vi "调制信号与解调.vi"() -> ()   [LabVIEW 2018]
panel:
  out "布尔":bool
  out "数组 2":dbl[](array[numeric])
  out "解调后的波形":dynamicdata(graph)
  out "相干后时域波形":dynamicdata(graph)
  in  "停止":bool
  out "数组":dbl[](array[numeric])
  in  "垂直指针滑动杆":dbl(slide) min=0.0 max=5.0 scale=0.0..5.0
  out "波形图":dynamicdata(graph)
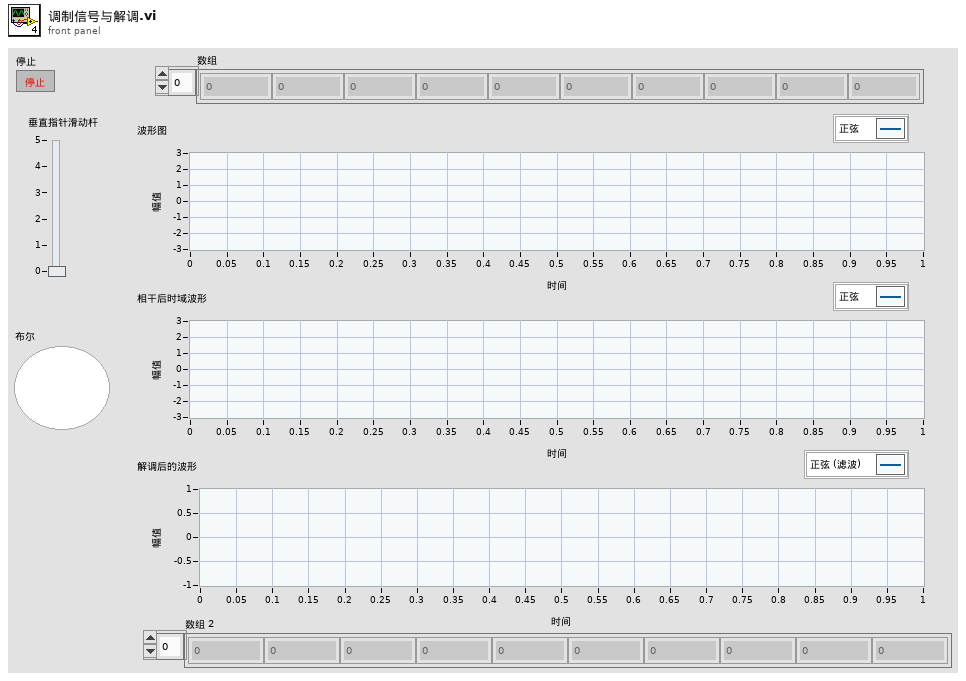
[diagram p1: front panel]
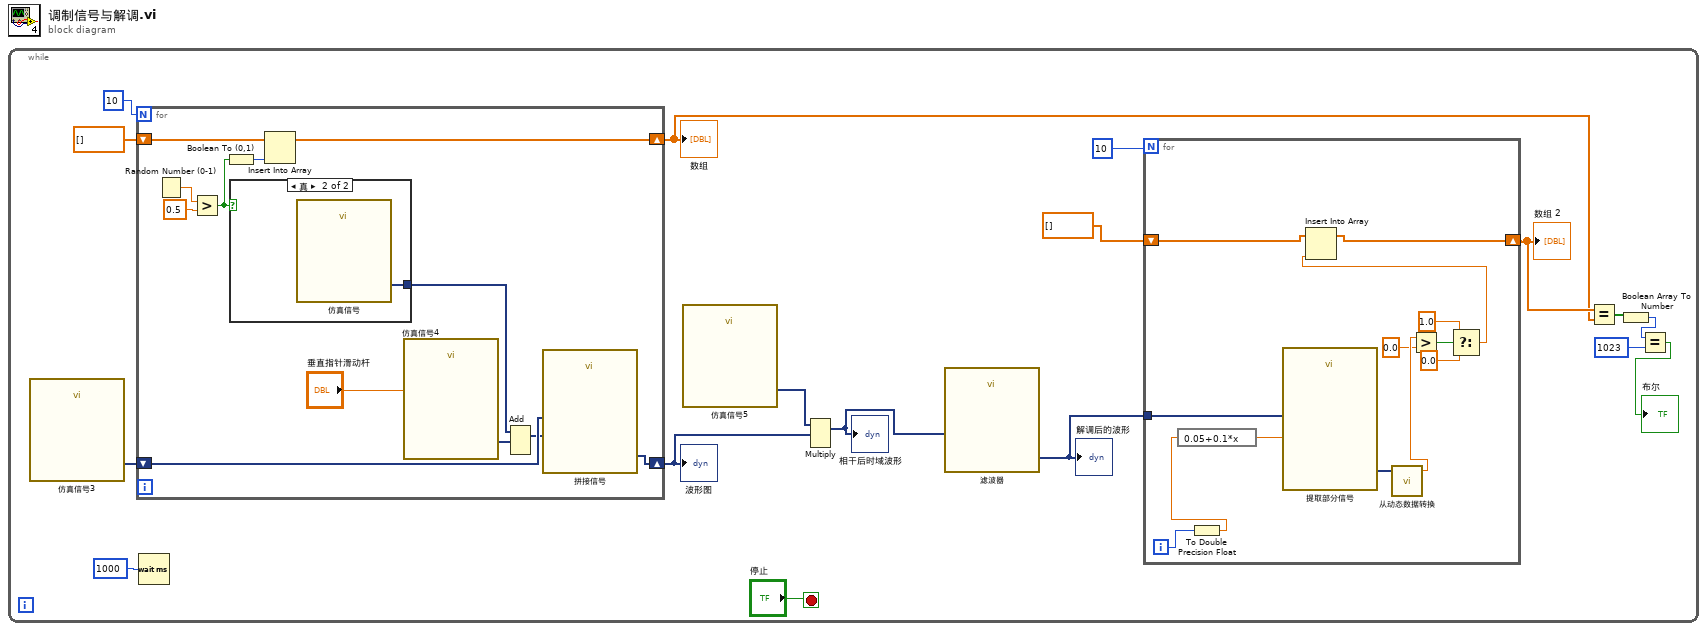
[diagram p0: block diagram]
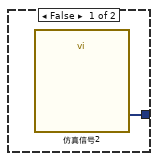
[diagram p2: hidden frame]
diagram:
  n1 = while {
    stop <- "停止" stop-if-true
    n2 = call "仿真信号3"() -> ("正弦"=w16:dynamicdata)  [unwired: 14 in, 1 out]
    n3 = for {
      N: 10 -> [_]
      shift-right: [w40] -> w11
      shift-left: w16 -> [w39]
      shift-right: [w31] -> w5
      shift-left: dbl[] [] -> [w34]
      n4 = Random Number (0-1)() -> (number: 0 to 1=w41:dbl)
      n5 = Greater?(x=w41, y=0.5) -> (0:w33:bool)
      n6 = Boolean To (0,1)(Boolean=w33) -> (0, 1=w32:i16)
      n7 = case shown="真" w33 {
        tunnel: [w43 w44] -> w37
        frame False {
          n8 = call "仿真信号2"() -> ("正弦"=w43:dynamicdata)  [unwired: 14 in, 1 out]
        }
        frame True {
          n9 = call "仿真信号"() -> ("正弦"=w44:dynamicdata)  [unwired: 14 in, 1 out]
        }
      }
      n10 = Insert Into Array(array=w34, new element=w32) -> (w31:dbl[])  [unwired: 1 in]
      n11 = call "仿真信号4"("噪声幅值"="垂直指针滑动杆") -> ("正弦与均匀噪声"=w36:dynamicdata)  [unwired: 13 in, 1 out]
      n12 = Add(1:w36, 2:w37) -> (0:w35:dynamicdata)  [unwired: 1 in, 1 out]
      n13 = call "拼接信号"("Input Signal B"=w35, "Input Signal A"=w39) -> ("Appended Signals"=w40:dynamicdata)  [unwired: 8 in, 1 out]
    }
    "波形图" <- w11
    "数组" <- w5
    n14 = Wait (ms)(milliseconds to wait=u32 1000 ("等待时间（毫秒）")) -> ()  [unwired: 1 out]
    n15 = call "仿真信号5"() -> ("正弦"=w12:dynamicdata)  [unwired: 14 in, 1 out]
    n16 = Multiply(1:w11, 2:w12) -> (0:w10:dynamicdata)  [unwired: 1 in, 1 out]
    "相干后时域波形" <- w10
    n17 = call "滤波器"("Signal"=w10) -> ("Filtered Signal"=w8:dynamicdata)  [unwired: 9 in, 1 out]
    "解调后的波形" <- w8
    n18 = for {
      N: 10 -> [_]
      tunnel: w8 -> [w29]
      shift-right: [w18] -> w6
      shift-left: dbl[] [] -> [w20]
      i -> [w27]
      n19 = To Double Precision Float(number=w27) -> (double precision float=w26:dbl)
      n20 = expression code="0.05+0.1*x"(w26) -> (w30:dbl)
      n21 = call "提取部分信号"("Begin Offset"=w30, "Signals"=w29) -> ("Section"=w28:dynamicdata)  [unwired: 8 in, 1 out]
      n22 = call "从动态数据转换"("Dynamic Data Type"=w28) -> ("Scalar"=w25:dbl)  [unwired: 3 in]
      n23 = Greater?(x=w25, y=0.0) -> (0:w23:bool)
      n24 = Select(t=1.0, s=w23, f=0.0) -> (s? t:f=w19:dbl)
      n25 = Insert Into Array(array=w20, new element=w19) -> (w18:dbl[])  [unwired: 1 in]
    }
    "数组 2" <- w6
    n26 = Equal?(x=w6, y=w5) -> (x = y?=w4:bool[])
    n27 = Boolean Array To Number(Boolean array=w4) -> (number=w3:u32)
    n28 = Equal?(x=w3, y=u32 1023) -> (x = y?=→"布尔":bool)
  }
